vi "TrendsD03.vi"() -> ()   [LabVIEW 2019, in "D03.lvlib"]
uses:
  D03.lvlib
  <vilib>/measure/mamon.llb/Trigger Detection for 1 Channel.vi
  <vilib>/measure/NI_MAPro.lvlib
panel:
  out "No Change":bool
  out "Sudden Change":bool
  out "Decrease":bool
  out "Increase":bool
  out "Previous  ES":dbl
  out "Present  Speed":dbl
  out "Present Error":dbl format="%#.2g"
  out "Previous Error":dbl
  out "Previous  Speed":dbl
  out "Previous PW":dbl caption="Control Information"
  out "Pulse Trends":waveform(i16)[](graph) caption="Waveform Chart - Dark"
  in  "Close":bool
  out "disc name":string="Disc 03 Trends"
  out "dsgs":string="DSGS"
  out "Speed Trend":waveform(dbl)(graph) caption="Waveform Chart - Dark"
  out "Average Trend":waveform(dbl)[](graph) caption="Waveform Chart - Dark"
  out "Live Trend":waveform(dbl)[](graph) caption="Waveform Chart - Dark"
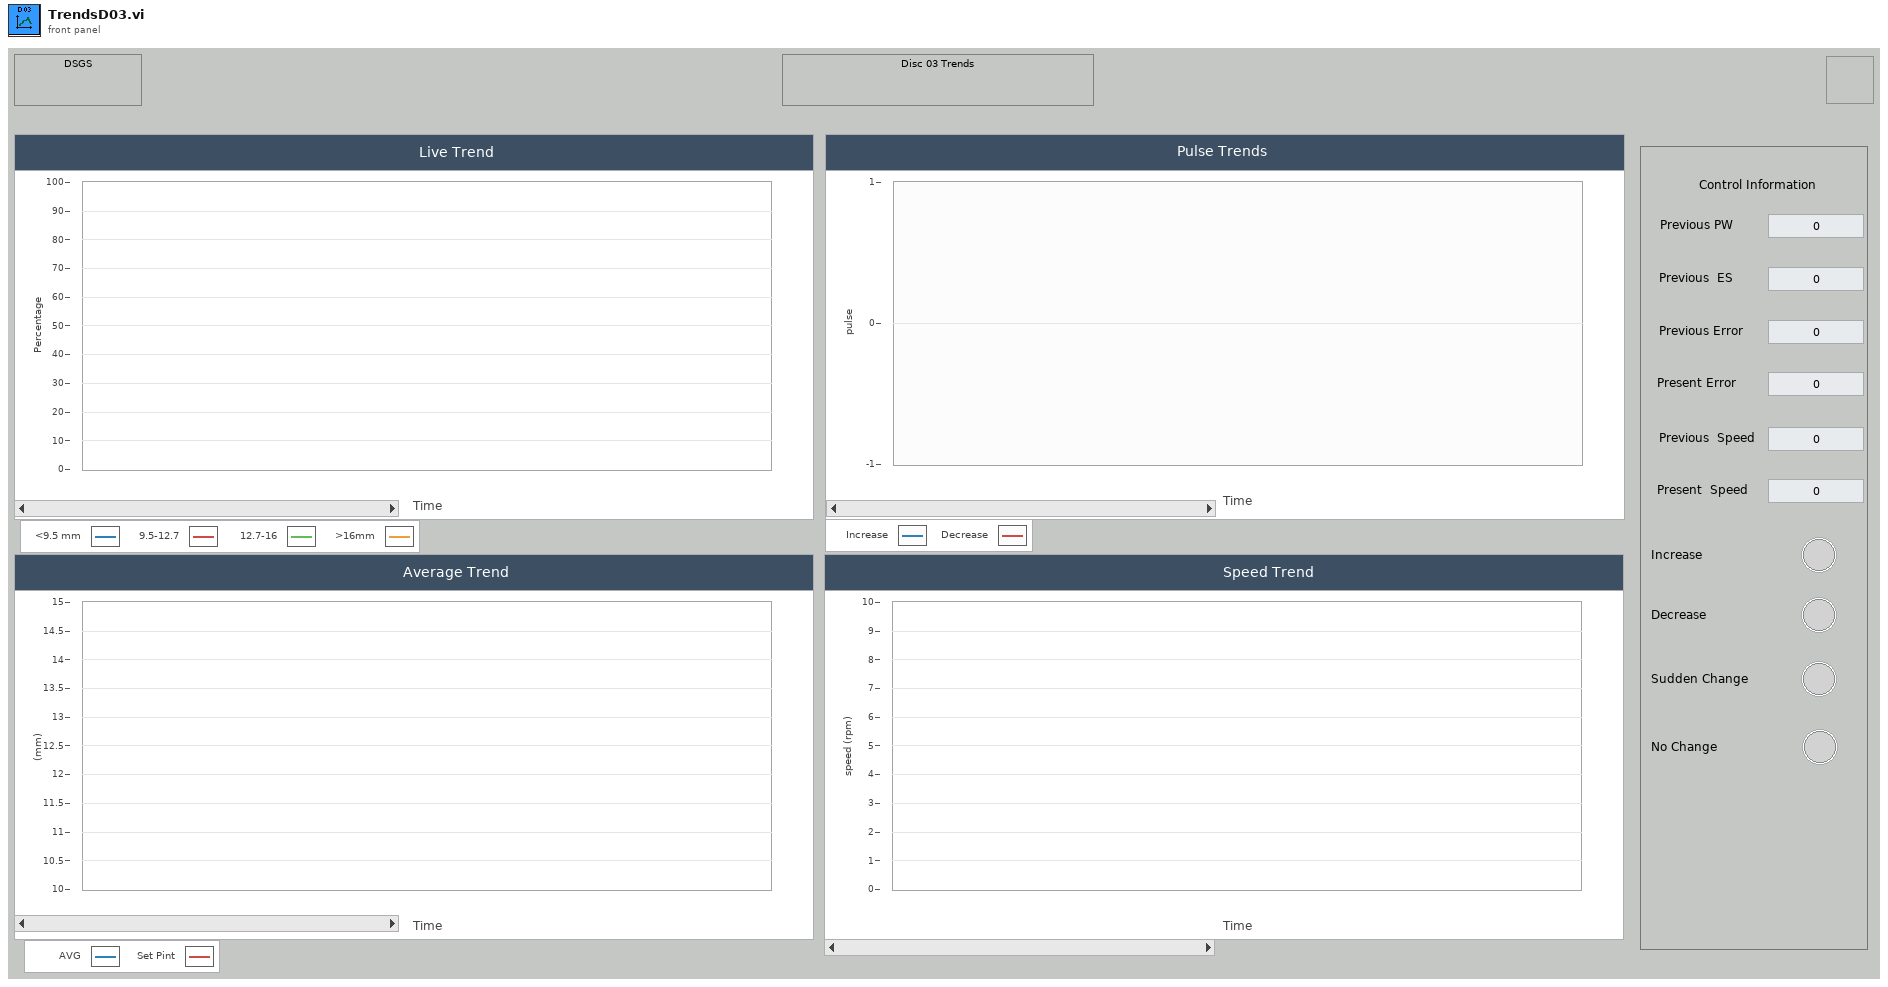
[diagram p1: front panel]
types:
  T1 = cluster{"decrease D03":bool, "increase D03":bool, "no change D03":bool, "sudden change D03":bool, "last error 03":dbl, "previous speed D03":dbl, "pulse width D03":dbl, "slope D03":dbl}
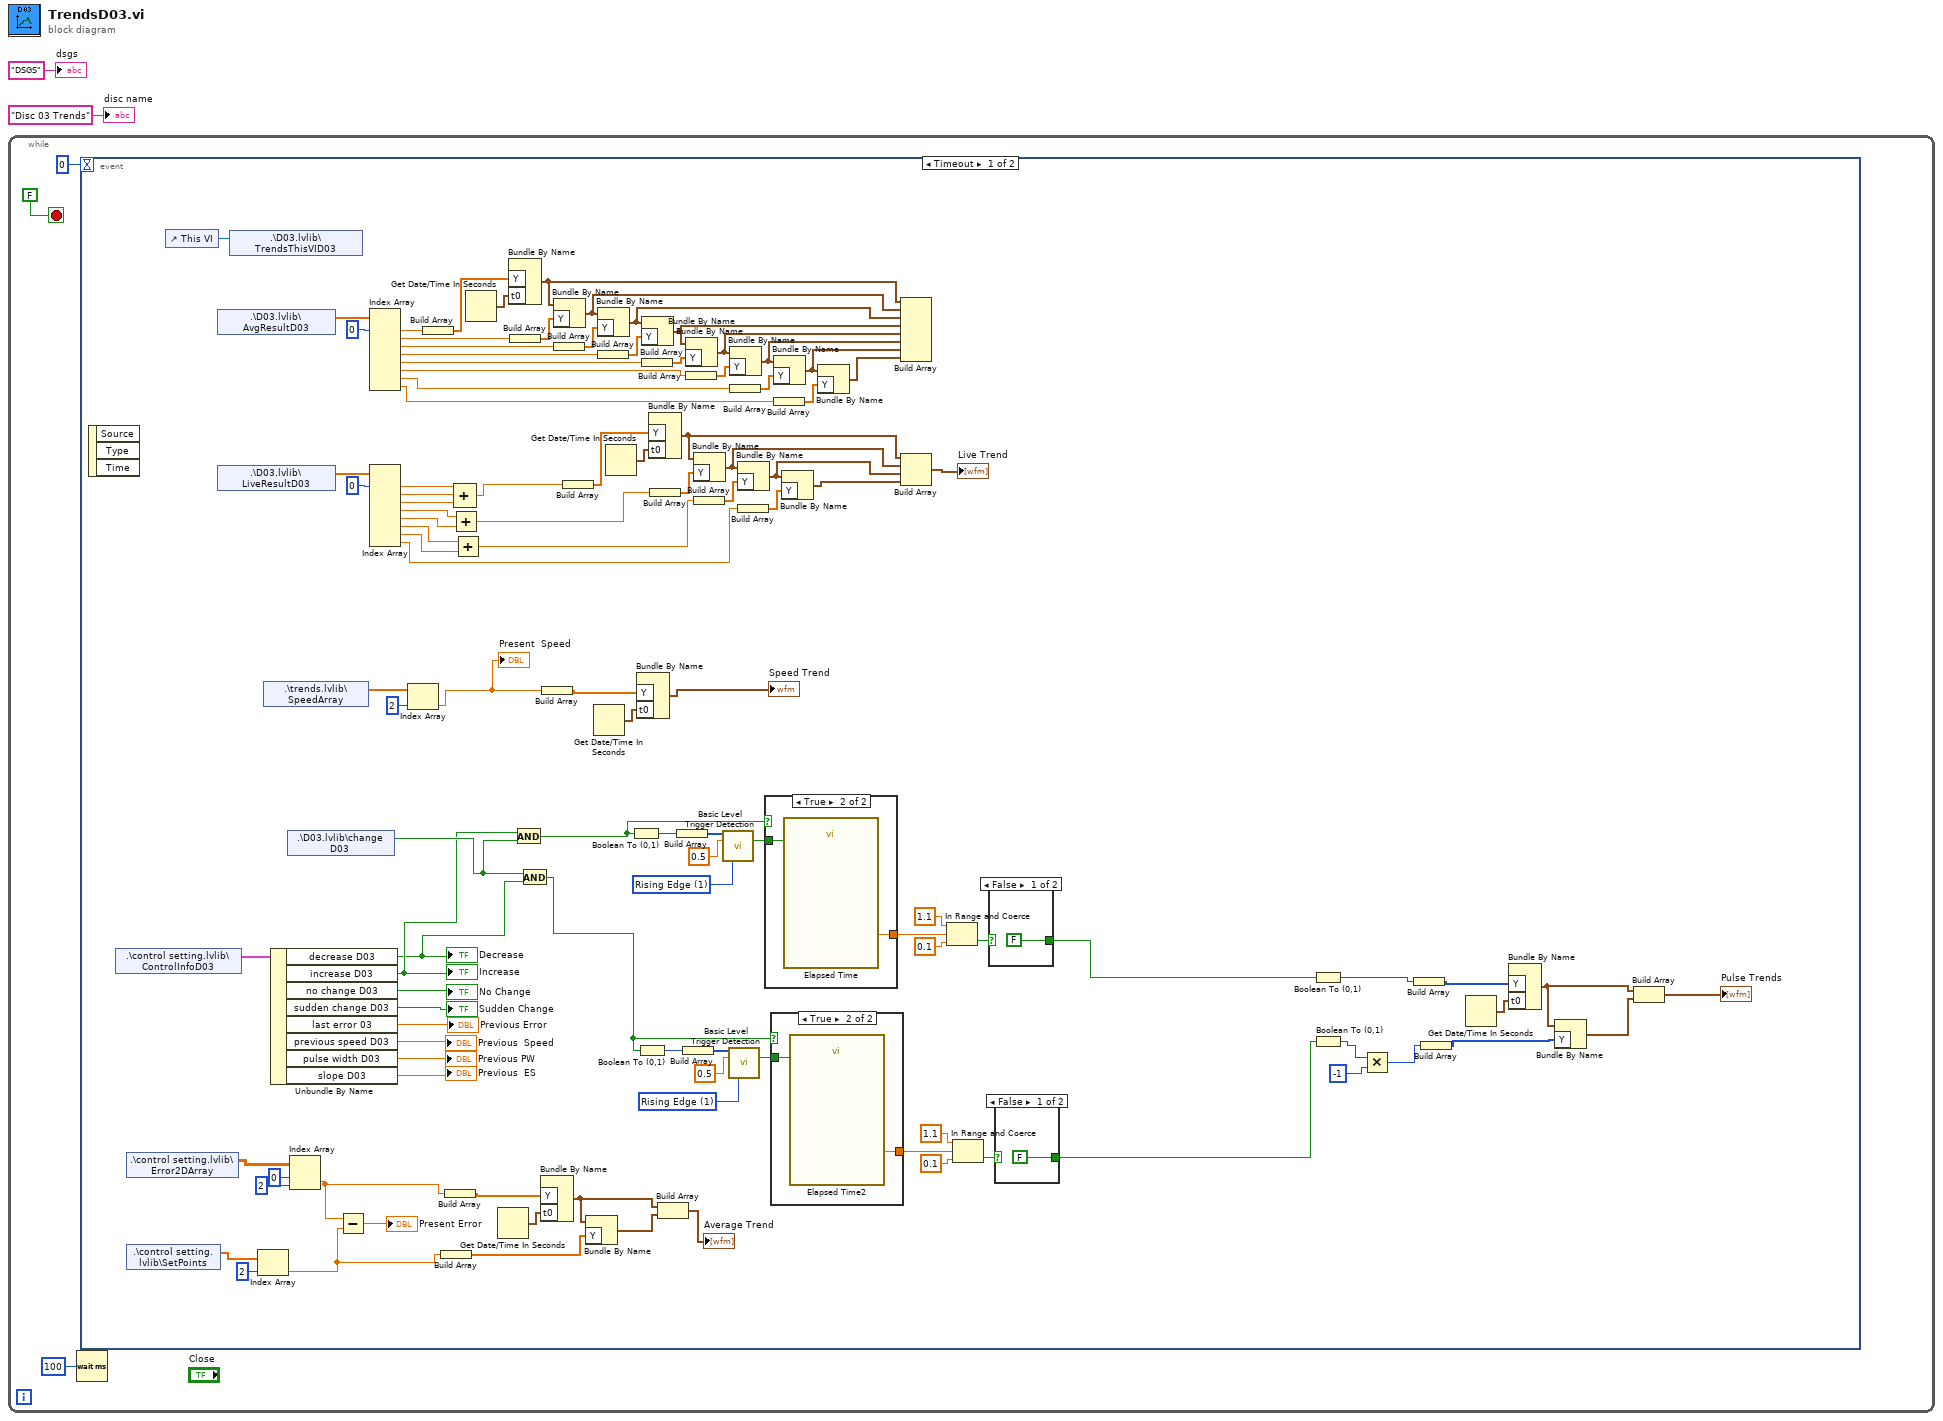
[diagram p0: block diagram]
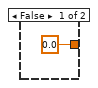
[diagram p2: hidden frame]
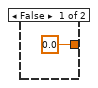
[diagram p4: hidden frame]
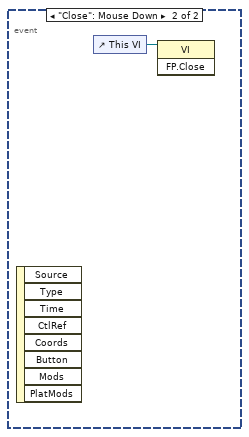
[diagram p6: hidden frame]
diagram:
  n1 = while {
    stop <- FALSE stop-if-true
    n2 = Wait (ms)(milliseconds to wait=u32 100) -> ()  [unwired: 1 out]
    n3 = event shown="[0] Timeout" {
      selector: _ -> [_ _]
      dyn-events: _ -> [_ _]
      timeout: 0 -> [_ _]
      event Timeout {
        w35 = u16 1 items=["Falling Edge", "Rising Edge"] ("trigger slope")
        w40 = u16 1 items=["Falling Edge", "Rising Edge"] ("trigger slope")
        n4 = event-data() -> ()  [unwired: 1 in, 3 out]
        n5 = shared-variable ".\\control setting.lvlib\\ControlInfoD03"() -> (w63:T1)  [unwired: 1 in, 1 out]
        n6 = shared-variable ".\\control setting.lvlib\\Error2DArray"() -> (w57:dbl[][])  [unwired: 1 in, 1 out]
        n7 = shared-variable ".\\control setting.lvlib\\SetPoints"() -> (w54:dbl[])  [unwired: 1 in, 1 out]
        n8 = control-ref of="This VI"() -> (w79:refnum<vi>)
        n9 = shared-variable ".\\D03.lvlib\\AvgResultD03"() -> (w85:dbl[])  [unwired: 1 in, 1 out]
        n10 = shared-variable ".\\D03.lvlib\\LiveResultD03"() -> (w118:dbl[])  [unwired: 1 in, 1 out]
        n11 = shared-variable ".\\D03.lvlib\\TrendsThisVID03"(w79) -> ()  [unwired: 1 in, 1 out]
        n12 = Index Array(array=w54, index=2) -> (element=w10:dbl)
        n13 = shared-variable ".\\trends.lvlib\\SpeedArray"() -> (w68:dbl[])  [unwired: 1 in, 1 out]
        n14 = Unbundle By Name(w63) -> ("decrease D03"=w27:bool, "increase D03"=w48:bool, "no change D03"=→"No Change":bool, "sudden change D03"=→"Sudden Change":bool, "last error 03"=→"Previous Error":dbl, "previous speed D03"=→"Previous  Speed":dbl, "pulse width D03"=→"Previous PW":dbl, "slope D03"=→"Previous  ES":dbl)
        "Increase" <- w48
        "Decrease" <- w27
        n15 = shared-variable ".\\D03.lvlib\\change D03"() -> (w49:bool)  [unwired: 1 in, 1 out]
        n16 = Index Array(array=w57, index (row)=0, index (col)=2 ("disabled index (col)")) -> (element=w12:dbl)
        n17 = Subtract(x=w12, y=w10) -> (x-y=→"Present Error":dbl)
        n18 = Index Array(array=w85, index #1=0 ("index")) -> (element #1=w95:dbl, element #2=w96:dbl, element #3=w98:dbl, element #4=w100:dbl, element #5=w101:dbl, element #6=w103:dbl, element #7=w105:dbl, element #8=w84:dbl)  [unwired: 7 in]
        n19 = Index Array(array=w118, index #1=0 ("index")) -> (element #1=w24:dbl, element #2=w23:dbl, element #3=w22:dbl, element #4=w21:dbl, element #5=w20:dbl, element #6=w19:dbl, element #7=w18:dbl, element #8=w14:dbl)  [unwired: 7 in]
        n20 = Index Array(array=w68, index=2) -> (element=w50:dbl)
        "Present  Speed" <- w50
        n21 = Build Array(w95) -> (w106:dbl[])
        n22 = Build Array(w10) -> (w9:dbl[])
        n23 = Build Array(w12) -> (w11:dbl[])
        n24 = Add(x=w21, y=w20) -> (x+y=w16:dbl)
        n25 = Add(x=w19, y=w18) -> (x+y=w15:dbl)
        n26 = Compound Arithmetic op=ADD(w24, w23, w22) -> (w17:dbl)
        n27 = Get Date/Time In Seconds() -> (seconds since 1Jan1904=w88:timestamp)
        n28 = Get Date/Time In Seconds() -> (seconds since 1Jan1904=w13:timestamp)
        n29 = Bundle By Name("Y"=w106, "t0"=w88) -> (w94:waveform(dbl))  [unwired: 1 in]
        n30 = Build Array(w96) -> (w97:dbl[])
        n31 = And(x=w48, y=w49) -> (x .and. y?=w38:bool)
        n32 = And(x=w49, y=w27) -> (x .and. y?=w25:bool)
        n33 = Bundle By Name("Y"=w11, "t0"=w13) -> (w8:waveform(dbl))  [unwired: 1 in]
        n34 = Build Array(w50) -> (w66:dbl[])
        n35 = Bundle By Name(cluster=w94, "Y"=w97) -> (w93:waveform(dbl))
        n36 = Build Array(w98) -> (w99:dbl[])
        n37 = Build Array(w17) -> (w108:dbl[])
        n38 = Bundle By Name(cluster=w8, "Y"=w9) -> (w7:waveform(dbl))
        n39 = Get Date/Time In Seconds() -> (seconds since 1Jan1904=w65:timestamp)
        n40 = Bundle By Name(cluster=w93, "Y"=w99) -> (w92:waveform(dbl))
        n41 = Build Array(w100) -> (w87:dbl[])
        n42 = Get Date/Time In Seconds() -> (seconds since 1Jan1904=w115:timestamp)
        n43 = Boolean To (0,1)(Boolean=w38) -> (0, 1=w43:i16)
        n44 = Bundle By Name("Y"=w66, "t0"=w65) -> (→"Speed Trend":waveform(dbl))  [unwired: 1 in]
        n45 = Boolean To (0,1)(Boolean=w25) -> (0, 1=w32:i16)
        n46 = Bundle By Name(cluster=w92, "Y"=w87) -> (w91:waveform(dbl))
        n47 = Build Array(w101) -> (w102:dbl[])
        n48 = Bundle By Name("Y"=w108, "t0"=w115) -> (w111:waveform(dbl))  [unwired: 1 in]
        n49 = Build Array(w16) -> (w110:dbl[])
        n50 = Build Array(w8, w7) -> (→"Average Trend":waveform(dbl)[])
        n51 = Build Array(w43) -> (w42:i16[])
        n52 = Build Array(w32) -> (w33:i16[])
        n53 = Bundle By Name(cluster=w91, "Y"=w102) -> (w90:waveform(dbl))
        n54 = Build Array(w103) -> (w104:dbl[])
        n55 = Bundle By Name(cluster=w111, "Y"=w110) -> (w112:waveform(dbl))
        n56 = Build Array(w15) -> (w109:dbl[])
        n57 = call-poly <vilib>:"Basic Level Trigger Detection.vi"("signal in"=w42, "level"=0.5, "trigger slope"=w40) -> ("trigger detected?"=w39:bool)  [unwired: 10 in, 2 out]
        n58 = call-poly <vilib>:"Basic Level Trigger Detection.vi"("signal in"=w33, "level"=0.5, "trigger slope"=w35) -> ("trigger detected?"=w36:bool)  [unwired: 10 in, 2 out]
        n59 = Bundle By Name(cluster=w90, "Y"=w104) -> (w89:waveform(dbl))
        n60 = Build Array(w105) -> (w107:dbl[])
        n61 = Bundle By Name(cluster=w112, "Y"=w109) -> (w113:waveform(dbl))
        n62 = Build Array(w14) -> (w116:dbl[])
        n63 = case shown="True" w38 {
          tunnel: [0.0 ("Elapsed Time (s)") w125] -> w47
          tunnel: w39 -> [_ w126]
          frame False {
          }
          frame True {
            n64 = call "Elapsed Time"("Reset"=w126) -> ("Elapsed Time (s)"=w125:dbl)  [unwired: 11 in, 7 out]
          }
        }
        n65 = case shown="True" w25 {
          tunnel: [0.0 ("Elapsed Time (s)") w120] -> w28
          tunnel: w36 -> [_ w121]
          frame False {
          }
          frame True {
            n66 = call "Elapsed Time2"("Reset"=w121) -> ("Elapsed Time (s)"=w120:dbl)  [unwired: 11 in, 7 out]
          }
        }
        n67 = Bundle By Name(cluster=w89, "Y"=w107) -> (w81:waveform(dbl))
        n68 = Build Array(w84) -> (w83:dbl[])
        n69 = Bundle By Name(cluster=w113, "Y"=w116) -> (w114:waveform(dbl))
        n70 = Bundle By Name(cluster=w81, "Y"=w83) -> (w82:waveform(dbl))
        n71 = Build Array(w94, w93, w92, w91, w90, w89, w81, w82) -> ()  [unwired: 1 out]
        n72 = Build Array(w111, w112, w113, w114) -> (→"Live Trend":waveform(dbl)[])
        n73 = In Range and Coerce(upper limit=1.1, x=w47, lower limit=0.1) -> (In Range?=w44:bool)  [unwired: 1 out]
        n74 = In Range and Coerce(upper limit=1.1, x=w28, lower limit=0.1) -> (In Range?=w31:bool)  [unwired: 1 out]
        n75 = case shown="False" w44 {
          selector: w44 -> [_ w128]
          tunnel: [FALSE w128] -> w37
          frame False {
          }
          frame True {
          }
        }
        n76 = case shown="False" w31 {
          selector: w31 -> [_ w123]
          tunnel: [FALSE w123] -> w26
          frame False {
          }
          frame True {
          }
        }
        n77 = Boolean To (0,1)(Boolean=w37) -> (0, 1=w76:i16)
        n78 = Boolean To (0,1)(Boolean=w26) -> (0, 1=w72:i16)
        n79 = Multiply(x=w72, y=i16 -1 ("0, 1")) -> (x*y=w70:i16)
        n80 = Build Array(w76) -> (w77:i16[])
        n81 = Build Array(w70) -> (w75:i16[])
        n82 = Get Date/Time In Seconds() -> (seconds since 1Jan1904=w78:timestamp)
        n83 = Bundle By Name("Y"=w77, "t0"=w78) -> (w74:waveform(i16))  [unwired: 1 in]
        n84 = Bundle By Name(cluster=w74, "Y"=w75) -> (w73:waveform(i16))
        n85 = Build Array(w74, w73) -> (→"Pulse Trends":waveform(i16)[])
      }
      event "Close": Mouse Down {
        n86 = event-data() -> ()  [unwired: 1 in, 8 out]
        n87 = control-ref of="This VI"() -> (w129:refnum<vi>)
        n88 = invoke class="VI" method="FP.Close"(reference=w129) -> ()  [unwired: 2 in, 3 out]
      }
    }
  }
  "dsgs" <- "DSGS" ("dsgs")
  "disc name" <- "Disc 03 Trends" ("disc name")
